vi "TimerHelper.vi"(0 "Start":bool, 5 "Pause/Resume":bool, 7 "Reset":bool, 9 "Stop":bool) -> (4 "Clock":dbl format="%#_6f")   [LabVIEW 2016]
doc: "This VI performs stopwatch function"
panel:
  # "STOPWATCH"
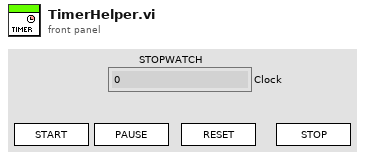
[diagram p1: front panel]
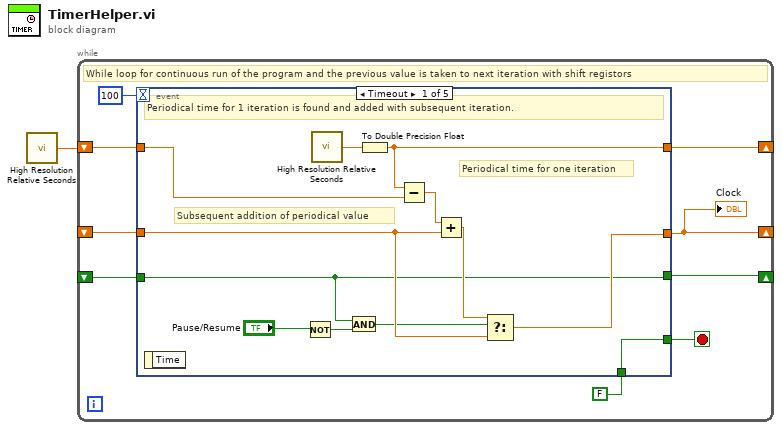
[diagram p0: block diagram]
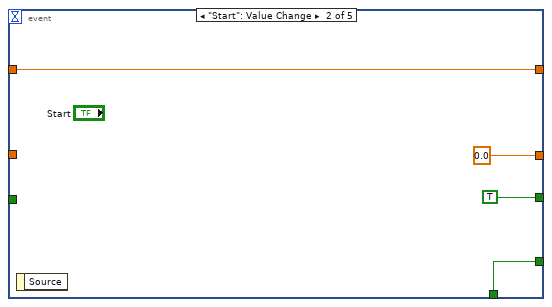
[diagram p2: hidden frame]
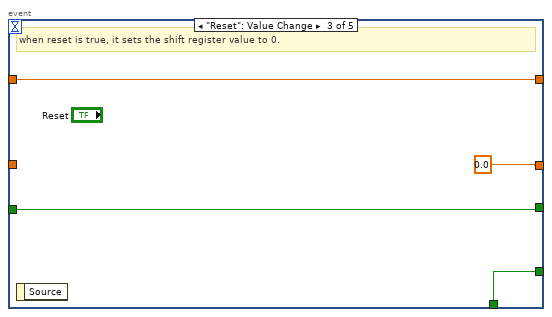
[diagram p3: hidden frame]
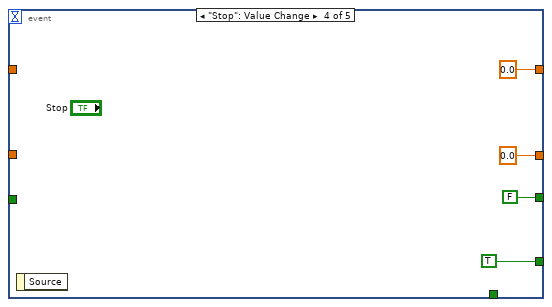
[diagram p4: hidden frame]
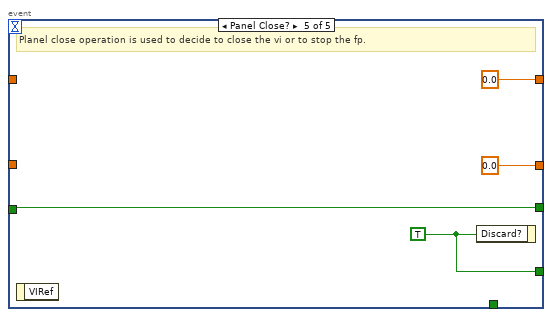
[diagram p5: hidden frame]
diagram:
  n1 = call <vilib>:"High Resolution Relative Seconds.vi"() -> ("relative seconds"=w1:dbl)
  n2 = while {
    shift-right: [w6] -> _
    shift-left: _ -> [w10]
    shift-right: [w9] -> _
    shift-left: w1 -> [w8]
    shift-right: [w5] -> _
    shift-left: _ -> [w4]
    stop <- w2 stop-if-true
    # "While loop for continuous run of the program and the previous value is taken to next iteration with shift registors"
    n3 = event shown="[0] Timeout" {
      selector: _ -> [_ _ _ _ _]
      dyn-events: _ -> [_ _ _ _ _]
      timeout: 100 -> [_ _ _ _ _]
      tunnel: w10 -> [w22 _ _ _ _]
      tunnel: [w21 w26 w30 0.0 ("relative seconds") 0.0 ("relative seconds")] -> w9
      tunnel: [w15 0.0 0.0 0.0 0.0] -> w6
      tunnel: w8 -> [w20 w26 w30 _ _]
      tunnel: w4 -> [w12 _ w28 _ w38]
      tunnel: [w12 TRUE w28 FALSE w38] -> w5
      tunnel: FALSE -> [w11 w23 w27 _ _]
      tunnel: [w11 w23 w27 TRUE w35] -> w2
      event Timeout {
        # "Subsequent addition of periodical value"
        # "Periodical time for one iteration"
        # "Periodical time for 1 iteration is found and added with subsequent iteration."
        n4 = event-data() -> ()  [unwired: 1 in, 1 out]
        n5 = Not(x="Pause/Resume") -> (.not. x?=w14:bool)
        n6 = call <vilib>:"High Resolution Relative Seconds.vi"() -> ("relative seconds"=w19:dbl)
        n7 = And(x=w12, y=w14) -> (x .and. y?=w13:bool)
        n8 = To Double Precision Float(number=w19) -> (double precision float=w21:dbl)
        n9 = Subtract(x=w21, y=w20) -> (x-y=w17:dbl)
        n10 = Add(x=w17, y=w22) -> (x+y=w18:dbl)
        n11 = Select(t=w18, s=w13, f=w22) -> (s? t:f=w15:dbl)
      }
      event "Start": Value Change {
        n12 = event-data() -> ()  [unwired: 1 in, 1 out]
      }
      event "Reset": Value Change {
        # "when reset is true, it sets the shift register value to 0."
        n13 = event-data() -> ()  [unwired: 1 in, 1 out]
      }
      event "Stop": Value Change {
        n14 = event-data() -> ()  [unwired: 1 in, 1 out]
      }
      event Panel Close? {
        w35 = TRUE
        # "Planel close operation is used to decide to close the vi or to stop the fp."
        n15 = event-data() -> ()  [unwired: 1 in, 1 out]
        n16 = event-data("Discard?"=w35) -> ()  [unwired: 1 in, 1 out]
      }
    }
    "Clock" <- w6
  }
